vi "Test MQTT-3.8.1-1.vi"(8 "error in (no error)":errorcluster) -> (0 "error out":errorcluster)   [LabVIEW 2013]
uses:
  source/Control Packets/SUBSCRIBE/Topic Subscription -- cluster.ctl
  source/Control Packets/ControlPacket/QualityOfService -- enum.ctl
  source/Control Packets/ControlPacket/ControlPacket.lvclass/ControlPacket.ctl
  source/Client/Client.lvclass
  <vilib>/addons/_JKI Toolkits/Caraya/classes/Test/Test.lvclass
  source/Control Packets/SUBSCRIBE/SUBSCRIBE.lvclass
  source/Control Packets/ControlPacket/ControlPacket.lvclass
  <vilib>/addons/_JKI Toolkits/Caraya/classes/Assert/Assert.lvclass
  source/MQTT_Base/MQTT_Base.lvclass
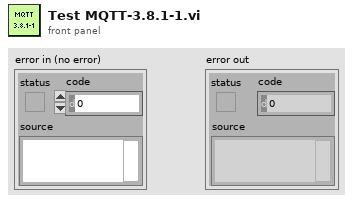
[diagram p1: front panel]
types:
  T1 = typedef "SUBSCRIBE.lvclass/Topic Subscription -- cluster.ctl" = cluster{"Topic Filter":string, "QoS":T2}
  T2 = typedef "ControlPacket.lvclass/QualityOfService -- enum.ctl" = enum16{"0 (At Most Once)", "1 (At Least Once)", "2 (Exactly Once)"}
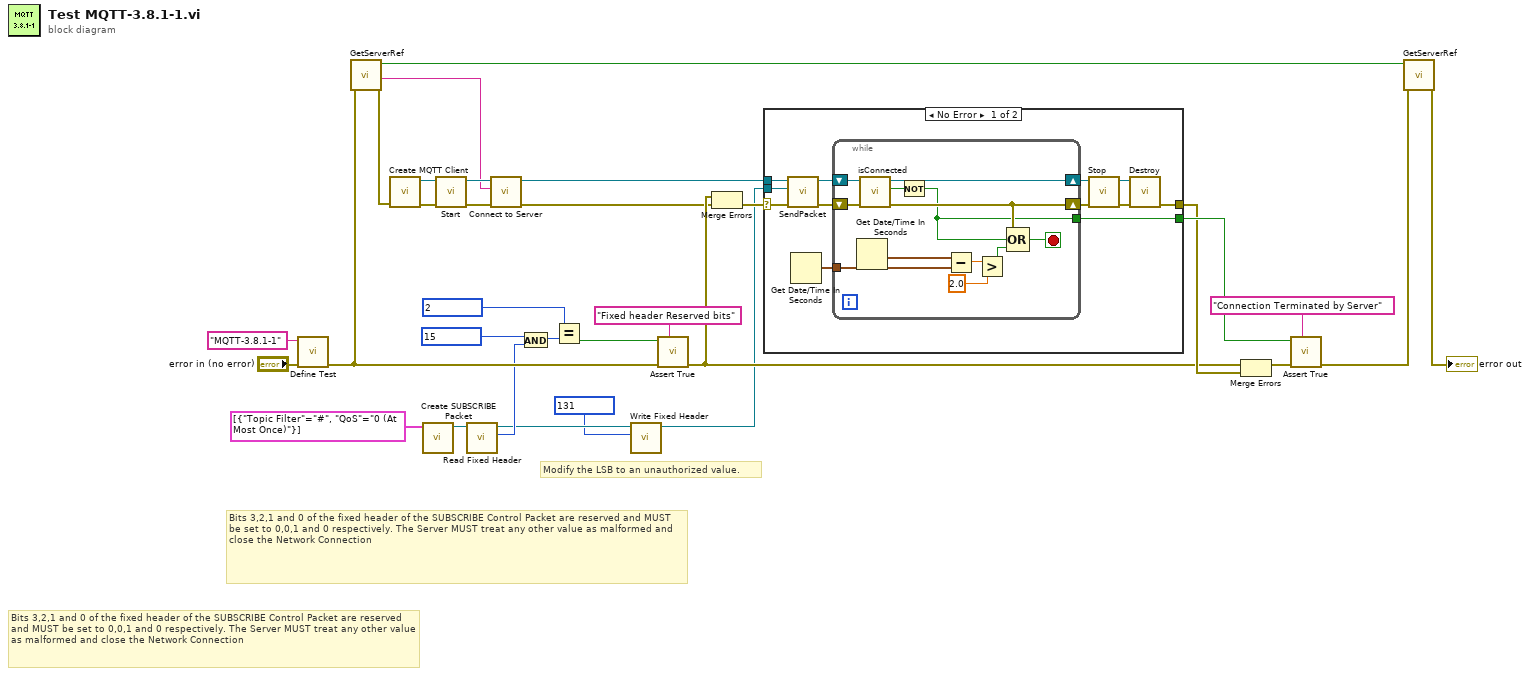
[diagram p0: block diagram]
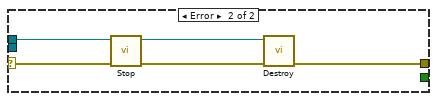
[diagram p2: hidden frame]
diagram:
  # "Modify the LSB to an unauthorized value."
  # "Bits 3,2,1 and 0 of the fixed header of the SUBSCRIBE Control Packet are reserved and MUST be set to 0,0,1 and 0 respectively. The Server MUST treat any other value as malformed and close the Network Connection"
  # "Bits 3,2,1 and 0 of the fixed header of the SUBSCRIBE Control Packet are reserved and MUST be set to 0,0,1 and 0 respectively. The Server MUST treat any other value as malformed and close the Network Connection"
  n1 = call <vilib>:"Define Test.vi"("error in (no error)"="error in (no error)", "Label (VI Title)"="MQTT-3.8.1-1") -> ("error out"=w20:errorcluster)  [unwired: 9 in]
  n2 = call "GetServerRef.vi"("error in"=w20) -> ("error out"=w28:errorcluster, "Server address"=w1:string, "Created"=w29:bool)  [unwired: 7 in, 1 out]
  n3 = call "Create MQTT Client.vi"("error in (no error)"=w28) -> ("error out"=w3:errorcluster, "Client out"=w5:refnum<class "Client.lvclass">)  [unwired: 9 in]
  n4 = call "Create SUBSCRIBE Packet.vi"("Topic Subscriptions"=T1[] [{"Topic Filter"="#", "QoS"=enum."0 (At Most Once)"}]) -> ("SUBSCRIBE out"=w23:refnum<class "SUBSCRIBE.lvclass">)  [unwired: 9 in, 1 out]
  n5 = call "Start.vi"("error in (no error)"=w3, "MQTT_Base in"=w5) -> ("error out"=w2:errorcluster, "MQTT_Base out"=w4:refnum<class "Client.lvclass">)  [unwired: 7 in, 1 out]
  n6 = call "Read Fixed Header.vi"("ControlPacket in"=w23) -> ("Fixed Header"=w15:u8, "ControlPacket out"=w10:refnum<class "SUBSCRIBE.lvclass">)  [unwired: 9 in]
  n7 = call "Connect to Server.vi"("error in (no error)"=w2, "address (localhost)"=w1, "Client in"=w4) -> ("error out"=w7:errorcluster, "Client out"=w6:refnum<class "Client.lvclass">)  [unwired: 5 in, 2 out]
  n8 = And(x=u8 15, y=w15) -> (x .and. y?=w13:u8)
  n9 = Equal?(x=u8 2, y=w13) -> (x = y?=w11:bool)
  n10 = call "Write Fixed Header.vi"("Fixed Header"=u8 131, "ControlPacket in"=w10) -> ("ControlPacket out"=w9:refnum<class "SUBSCRIBE.lvclass">)  [unwired: 9 in]
  n11 = call <vilib>:"Assert True.vi"("Label"="Fixed header Reserved bits", "error in (no error)"=w20, "True?"=w11) -> ("error out"=w17:errorcluster)  [unwired: 8 in]
  n12 = Merge Errors(w17, w7) -> (w16:errorcluster)
  n13 = case shown="No Error" w16 {
    selector: w16 -> [w41 w57]
    tunnel: w6 -> [w42 w59]
    tunnel: [w43 w60] -> w18
    tunnel: [w33 _] -> w24
    tunnel: w9 -> [w40 _]
    frame No Error {
      n14 = call "SendPacket.vi"("error in (no error)"=w41, "ControlPacket"=w40, "Client in"=w42) -> ("error out"=w36:errorcluster, "Client out"=w37:refnum<class "Client.lvclass">)  [unwired: 6 in, 1 out]
      n15 = Get Date/Time In Seconds() -> (seconds since 1Jan1904=w32:timestamp)
      n16 = while {
        shift-right: [w52] -> w35
        shift-left: w36 -> [w53]
        shift-right: [w54] -> w34
        shift-left: w37 -> [w55]
        tunnel: [w49] -> w33
        tunnel: w32 -> [w44]
        stop <- w51 stop-if-true
        n17 = Get Date/Time In Seconds() -> (seconds since 1Jan1904=w45:timestamp)
        n18 = call "isConnected.vi"("error in (no error)"=w53, "Client in"=w55) -> ("error out"=w52:errorcluster, "connected"=w50:bool, "Client out"=w54:refnum<class "Client.lvclass">)  [unwired: 7 in]
        n19 = Not(x=w50) -> (.not. x?=w49:bool)
        n20 = Subtract(x=w45, y=w44) -> (x-y=w48:dbl)
        n21 = Greater?(x=w48, y=2.0) -> (0:w46:bool)
        n22 = Compound Arithmetic op=OR(w52, w49, w46) -> (w51:bool)
      }
      n23 = call "Stop.vi"("error in (no error)"=w35, "MQTT_Base in"=w34) -> ("error out"=w38:errorcluster, "MQTT_Base out"=w39:refnum<class "Client.lvclass">)  [unwired: 7 in, 1 out]
      n24 = call-dynamic "Destroy.vi"("error in (no error)"=w38, "MQTT_Base in"=w39) -> ("error out"=w43:errorcluster)  [unwired: 8 in, 1 out]
    }
    frame Error {
      n25 = call "Stop.vi"("error in (no error)"=w57, "MQTT_Base in"=w59) -> ("error out"=w56:errorcluster, "MQTT_Base out"=w58:refnum<class "Client.lvclass">)  [unwired: 7 in, 1 out]
      n26 = call-dynamic "Destroy.vi"("error in (no error)"=w56, "MQTT_Base in"=w58) -> ("error out"=w60:errorcluster)  [unwired: 8 in, 1 out]
    }
  }
  n27 = Merge Errors(w17, w18) -> (w19:errorcluster)
  n28 = call <vilib>:"Assert True.vi"("Label"="Connection Terminated by Server", "error in (no error)"=w19, "True?"=w24) -> ("error out"=w27:errorcluster)  [unwired: 8 in]
  n29 = call "GetServerRef.vi"("error in"=w27, "Destroy (F)"=w29) -> ("error out"=→"error out":errorcluster)  [unwired: 6 in, 3 out]
